vi "Example_Single_Measurement_Main_v1.vi"() -> ()   [LabVIEW 2021]
uses:
  Config_File_Paths.ctl
panel:
  out "XY Graph 2":cluster{"Time":dbl[], "X":dbl[]}[](graph)
  out "Possible Mismatch In Phase (?)":bool
  out "Enough Points (?)":bool
  out "Trig Out Found(?)":bool
  out "XY Graph":cluster{"Time":dbl[], "X":dbl[]}[](graph)
  out "error out":errorcluster
  in  "Time unit":string(combo)="ms"
  in  "Config files paths":T1={"ZI config file (.ini)"="Config_Ver_1\\Zurich_params.ini", "Keithley config file (.ini)"="Config_Ver_1\\Keithley_params.ini", "Arduino config file (.ini)"="Config_Ver_1\\pulse_sequence.ini"}
  in  "error in":errorcluster
  in  "Resource Address":T2={"ZI Address"="DEV714", "VISA Keithley"="", "VISA Arduino PG"=""}
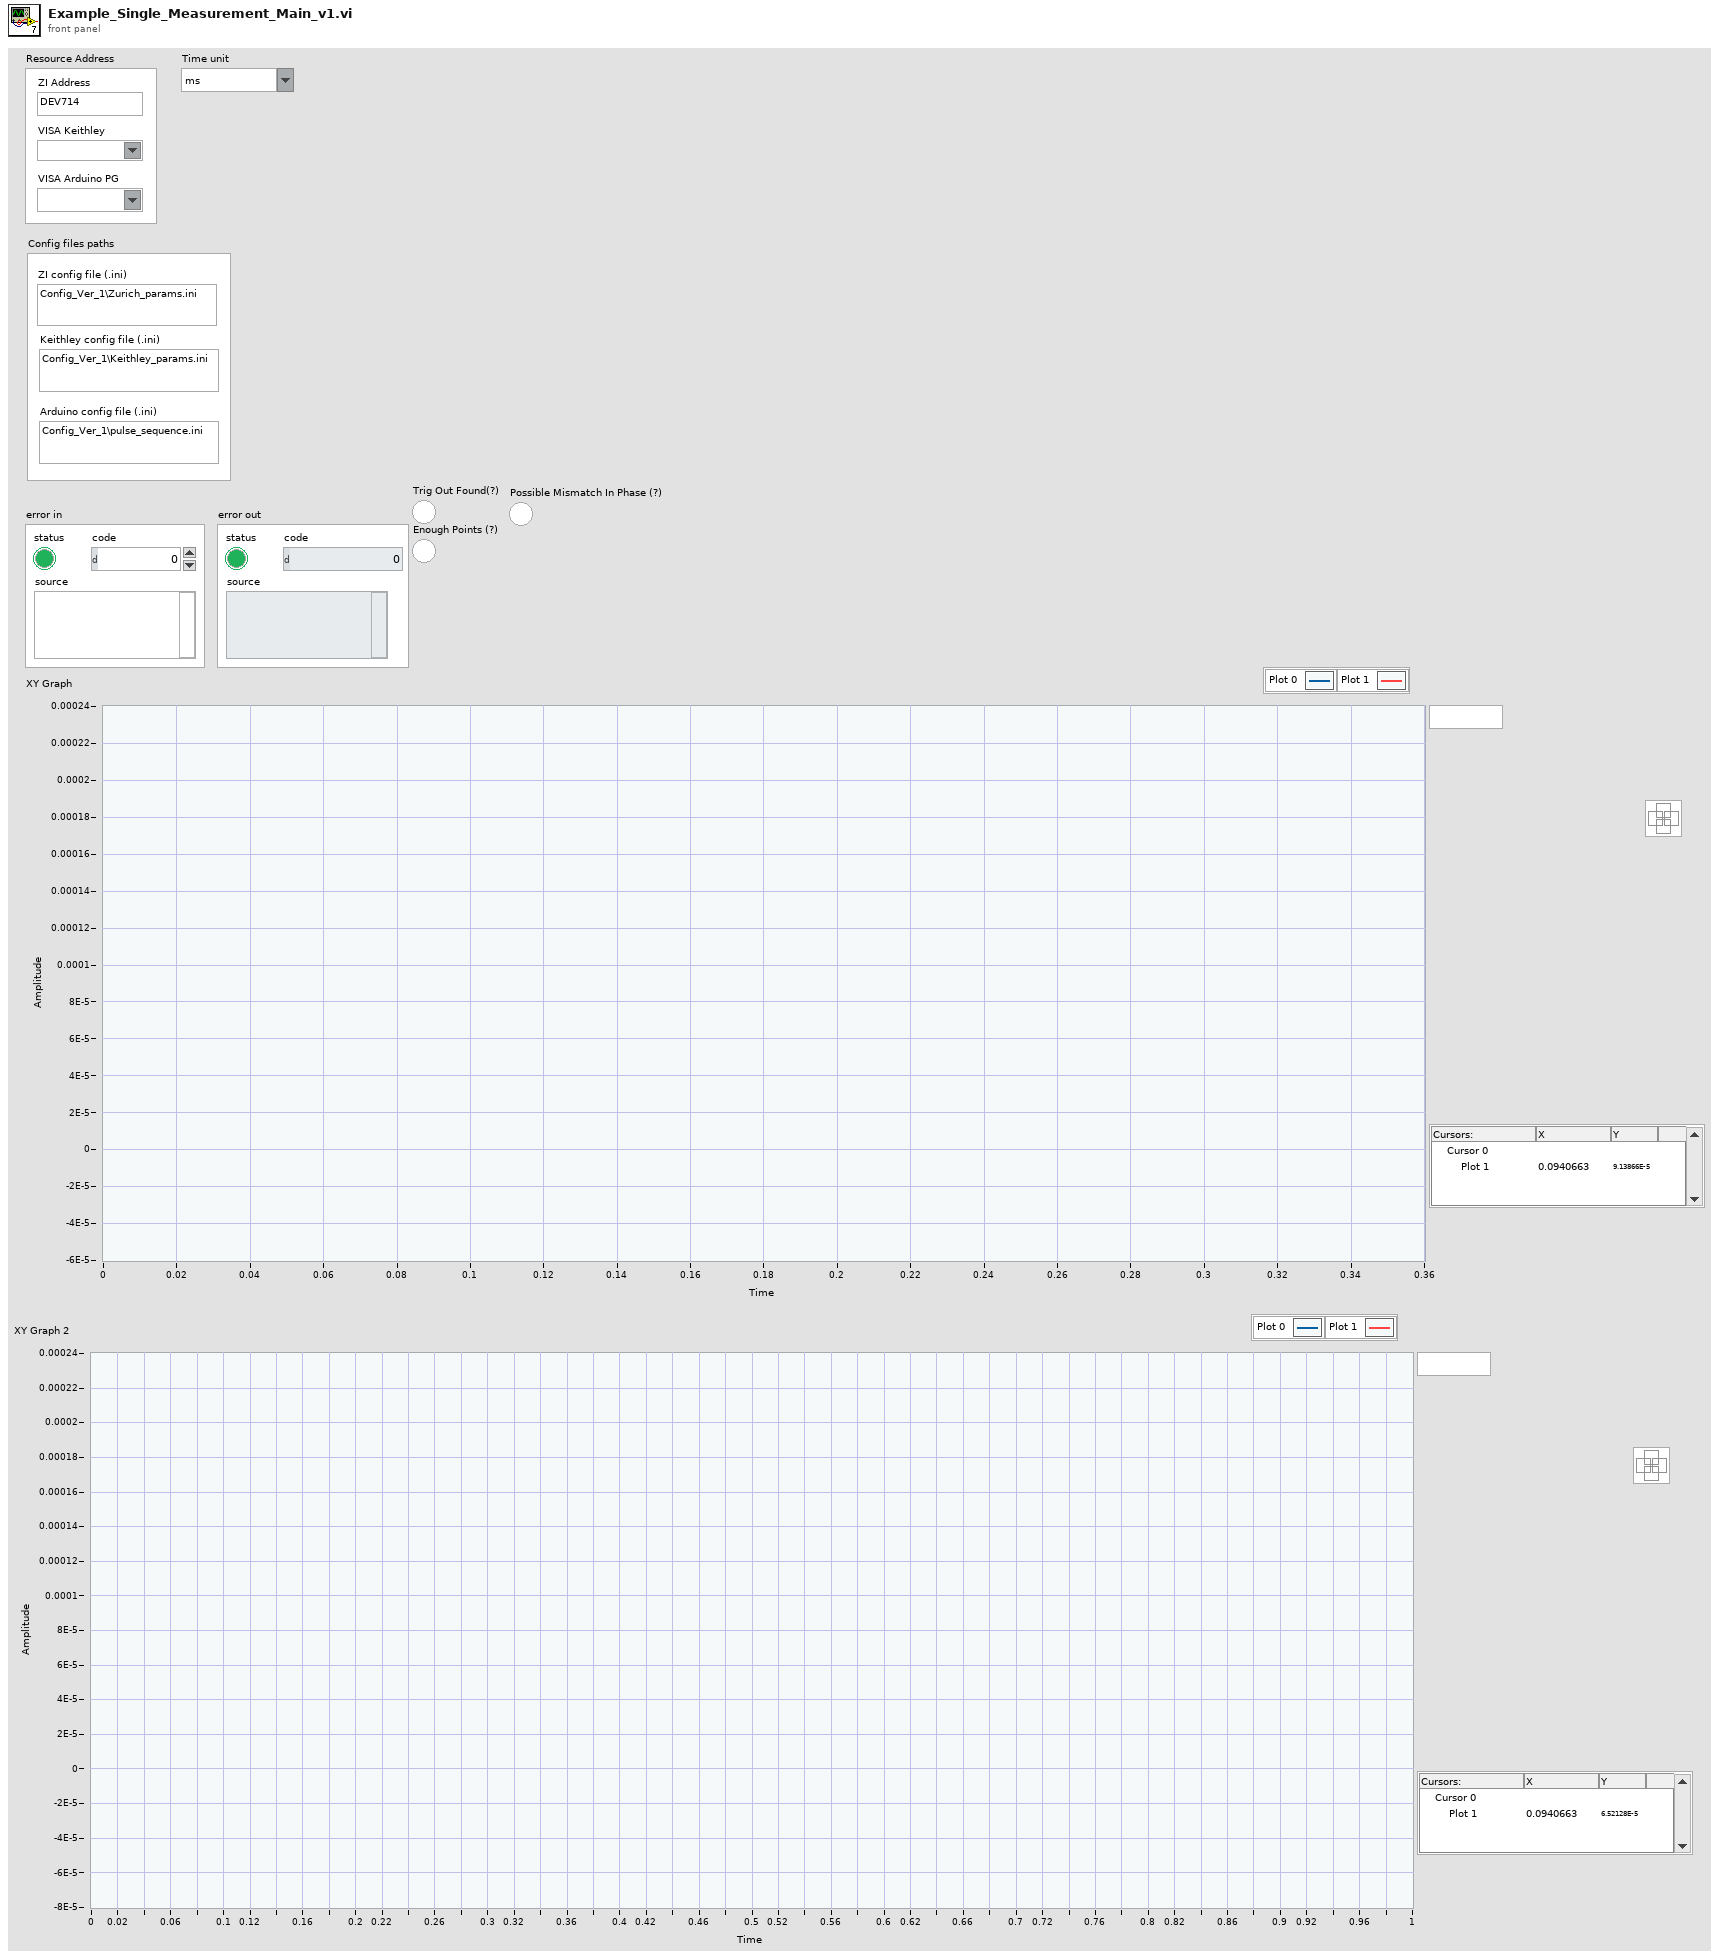
[diagram p1: front panel]
types:
  T1 = typedef "Config_File_Paths.ctl" = cluster{"ZI config file (.ini)":string, "Keithley config file (.ini)":string, "Arduino config file (.ini)":string}
  T2 = cluster{"ZI Address":string, "VISA Keithley":refnum<visa-resource-name>, "VISA Arduino PG":refnum<visa-resource-name>}
  T3 = typedef "Resources.ctl" = cluster{"ZI Handle":T4, "ZI ModHandle":T5, "VISA arduino":refnum<visa-resource-name>, "VISA Keithley":refnum<visa-resource-name>}
  T4 = typedef "Zurich Instruments LabOne.lvlib/ziTypeHandle.ctl" = cluster{"handleValid":bool, "Conn":u64, "Path Prefix":string, "Handle":u64, "Connected":bool, "Clockbase(s)":dbl}
  T5 = typedef "Zurich Instruments LabOne.lvlib/ziTypeModHandle.ctl" = cluster{"handleValid":bool, "Conn":u64, "ModHandle":u64, "moduleID":string, "Path Prefix":string}
  T6 = typedef "ZI_Data.ctl" = cluster{"R":dbl[], "Theta":dbl[], "X":dbl[], "Y":dbl[], "AuxIn0":dbl[], "AuxIn1":dbl[], "Frequency":dbl[], "DIO":dbl[], "Time":dbl[]}
  T7 = typedef "Cutted_Data.ctl" = cluster{"X":dbl[], "Y":dbl[], "Time":dbl[]}
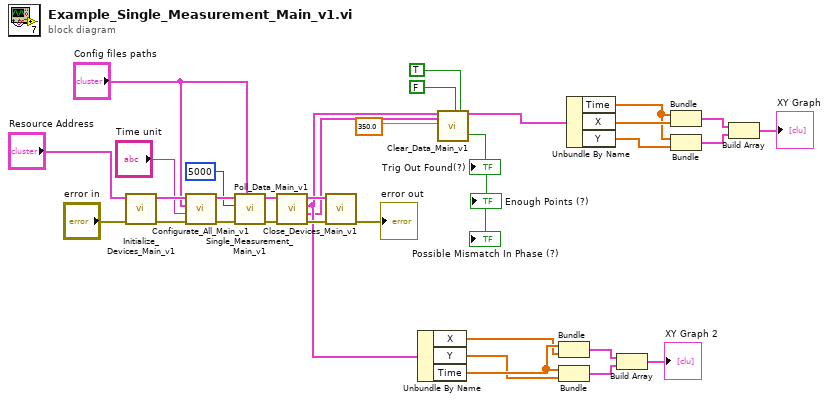
[diagram p0: block diagram]
diagram:
  n1 = call "Initialize_Devices_Main_v1.vi"("error in"="error in", "Resource Address"="Resource Address") -> ("error out"=w32:errorcluster, "Resources"=w33:T3)  [unwired: 8 in]
  n2 = call "Configurate_All_Main_v1.vi"("error in"=w32, "Time unit"="Time unit", "Config files paths"="Config files paths", "Resources in"=w33) -> ("error out"=w29:errorcluster, "Resources out"=w30:T3)  [unwired: 4 in, 2 out]
  n3 = call "Single_Measurement_Main_v1.vi"("Config files paths"="Config files paths", "error in"=w29, "Timeout [ms]"=u64 5000, "Resources In"=w30) -> ("error out"=w25:errorcluster, "Resources Out"=w26:T3)  [unwired: 6 in]
  n4 = call "Poll_Data_Main_v1.vi"("error in"=w25, "Resources in"=w26) -> ("error out"=w23:errorcluster, "ZI Data 3"=w6:T6, "ZI Data 0"=w13:T6, "Resources out"=w24:T3)  [unwired: 6 in]
  n5 = call "Close_Devices_Main_v1.vi"("error in"=w23, "Resources in"=w24) -> ("error out"=→"error out":errorcluster)  [unwired: 9 in]
  n6 = Unbundle By Name(w13) -> ("X"=w8:dbl[], "Y"=w7:dbl[], "Time"=w9:dbl[])
  n7 = call "Clear_Data_Main_v1.vi"("ZI Data 0"=w13, "ZI Data 3"=w6, "Time Of Collected Data (ms)"=350.0, "Fixed Number Of Points"=FALSE, "Check Phase Mismatch"=TRUE) -> ("Trig Out Found(?)"=→"Trig Out Found(?)":bool, "Enough Points (?)"=→"Enough Points (?)":bool, "Possible Mismatch In Phase (?)"=→"Possible Mismatch In Phase (?)":bool, "Cutted Data"=w4:T7)  [unwired: 9 in, 2 out]
  n8 = Bundle("Time"=w9, "X"=w8) -> (w10:cluster{"Time":dbl[], "X":dbl[]})  [unwired: 1 in]
  n9 = Bundle("Time"=w9, "Y"=w7) -> (w11:cluster{"Time":dbl[], "Y":dbl[]})  [unwired: 1 in]
  n10 = Unbundle By Name(w4) -> ("Time"=w1:dbl[], "X"=w3:dbl[], "Y"=w2:dbl[])
  n11 = Build Array(w10, w11) -> (→"XY Graph 2":cluster{"Time":dbl[], "Y":dbl[]}[])
  n12 = Bundle("Time"=w1, "X"=w3) -> (w21:cluster{"Time":dbl[], "X":dbl[]})  [unwired: 1 in]
  n13 = Bundle("Time"=w1, "Y"=w2) -> (w20:cluster{"Time":dbl[], "Y":dbl[]})  [unwired: 1 in]
  n14 = Build Array(w21, w20) -> (→"XY Graph":cluster{"Time":dbl[], "Y":dbl[]}[])
